vi "Build Actual View.vi"(5 "Encoder Counts Out":dbl[](array[numeric]), 7 "Speeds":dbl[](array[numeric]), 10 "Previous Actual":T5 {"Back Right"."Direction" scale format="%.3f"; "Back Right"."Velocity" format="%.2f"; "Back Left"."Direction" scale format="%.3f"; "Back Left"."Velocity" format="%.2f"; "Front Left"."Direction" scale format="%.3f"; "Front Left"."Velocity" format="%.2f"; "Front Right"."Direction" scale format="%.3f"; "Front Right"."Velocity" format="%.2f"}, 11 "Swerve Set":T1 {"Back Right"."Angle" scale format="%.3f"; "Back Right"."Velocity" scale=-1.0..1.0 scale format="%.1f"; "Back Left"."Angle" scale format="%.3f"; "Back Left"."Velocity" scale=-1.0..1.0 scale format="%.1f"; "Front Left"."Angle" scale format="%.3f"; "Front Left"."Velocity" scale=-1.0..1.0 scale format="%.1f"; "Front Right"."Angle" scale format="%.3f"; "Front Right"."Velocity" scale=-1.0..1.0 scale format="%.1f"}) -> (3 "Swerve Data out":T5 {"Back Right"."Direction" scale format="%.3f"; "Back Right"."Velocity" format="%.2f"; "Back Left"."Direction" scale format="%.3f"; "Back Left"."Velocity" format="%.2f"; "Front Left"."Direction" scale format="%.3f"; "Front Left"."Velocity" format="%.2f"; "Front Right"."Direction" scale format="%.3f"; "Front Right"."Velocity" format="%.2f"})   [LabVIEW 2020, in "SwerveDrive_ACT.lvlib"]
uses:
  SwerveDrive_ACT.lvlib
  Shared Code/TypeDefs/Cluster_Swerve Actual Settings.ctl
  Shared Code/TypeDefs/Cluster_Module Actual Settings.ctl
  Shared Code/TypeDefs/Dial_Actual Direction.ctl
  Shared Code/TypeDefs/Cluster_Swerve 4 Steer and Velocity.ctl
  Shared Code/TypeDefs/Cluster_Module Velocity-Direction-Rotations.ctl
  Shared Code/TypeDefs/Level_Velocity plus-minus 1.ctl
  Shared Code/TypeDefs/Dial_Compase heading unit circle CCW positive.ctl
panel:
  # "\"Front\" of Robot"
  # "Right Hand Rule"
  # "X"
  # "+CCW"
  # "Y"
  # "(0,0)"
  # "\"Front\" of Robot"
  # "X"
  # "+CCW"
  # "Y"
  # "(0,0)"
  # "\"Front\" of Robot"
  # "X"
  # "+CCW"
  # "Y"
  # "(0,0)"
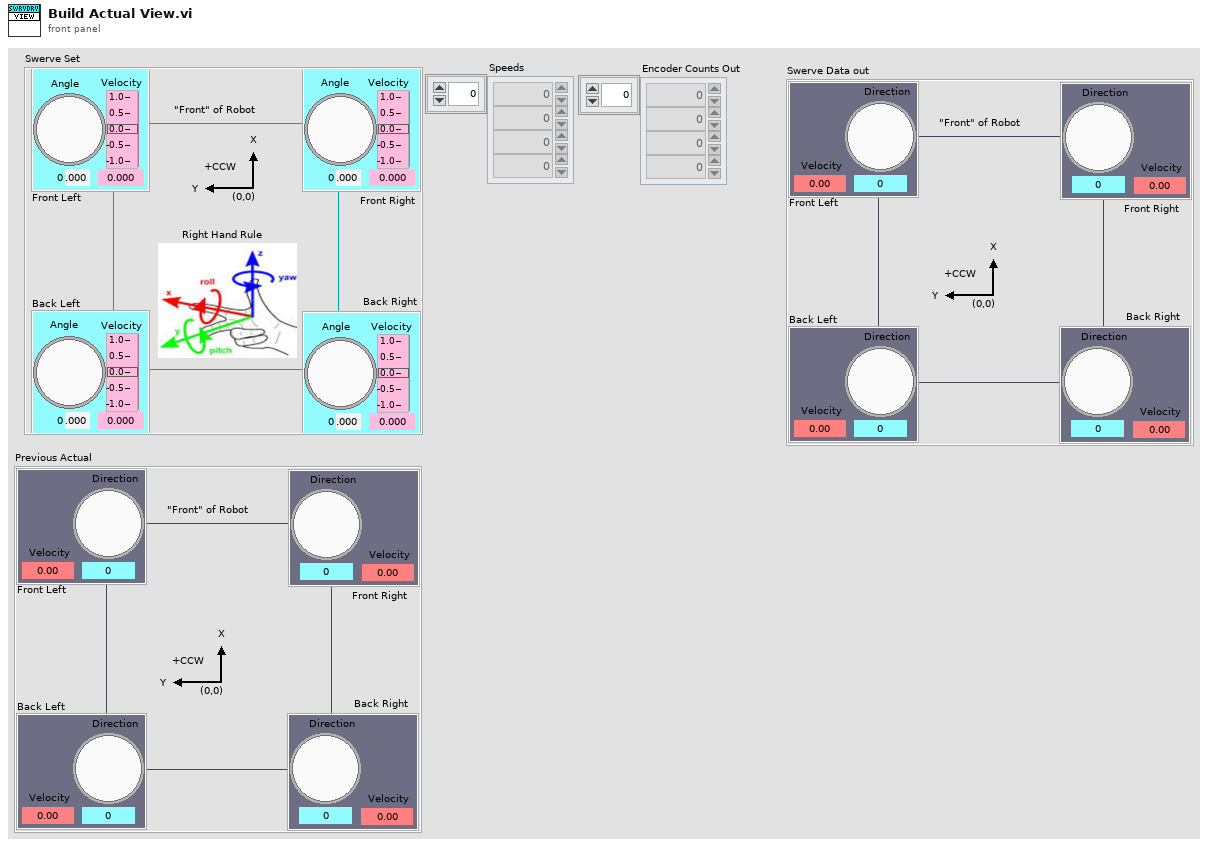
[diagram p1: front panel]
types:
  T1 = typedef "Cluster_Swerve 4 Steer and Velocity.ctl" = cluster{"Front Right":T2, "Front Left":T2, "Back Left":T2, "Back Right":T2}
  T2 = typedef "Cluster_Module Velocity-Direction-Rotations.ctl" = cluster{"Velocity":T3, "Angle":T4, "Rotations Count":dbl}
  T3 = typedef "Level_Velocity plus-minus 1.ctl" = dbl
  T4 = typedef "Dial_Compase heading unit circle CCW positive.ctl" = dbl
  T5 = typedef "Cluster_Swerve Actual Settings.ctl" = cluster{"Front Right":T6, "Front Left":T6, "Back Left":T6, "Back Right":T6}
  T6 = typedef "Cluster_Module Actual Settings.ctl" = cluster{"Velocity":dbl, "Direction":T7, "Encoder":dbl}
  T7 = typedef "Dial_Actual Direction.ctl" = dbl
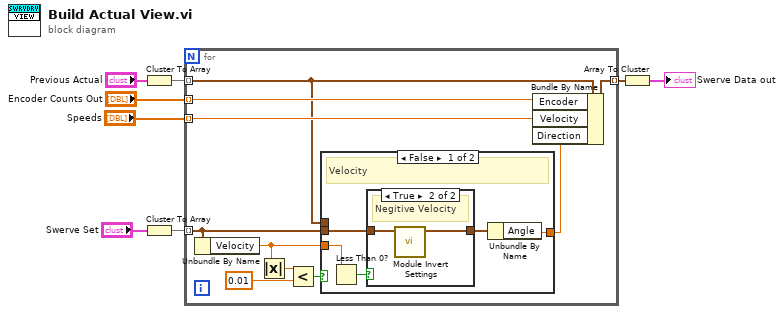
[diagram p0: block diagram]
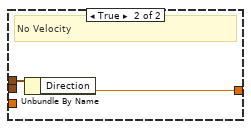
[diagram p3: hidden frame]
diagram:
  n1 = Cluster To Array(cluster="Previous Actual") -> (array=w6:T6[])
  n2 = Cluster To Array(cluster="Swerve Set") -> (array=w5:T2[])
  n3 = for {
    tunnel: w6 -> [w12] mode=indexing
    tunnel: w5 -> [w10] mode=indexing
    tunnel: "Encoder Counts Out" -> [w18] mode=indexing
    tunnel: "Speeds" -> [w16] mode=indexing
    tunnel: [w17] -> w2 mode=indexing
    n4 = Unbundle By Name(w10) -> ("Velocity"=w9:T3)
    n5 = Absolute Value(x=w9) -> (abs(x)=w15:T3)
    n6 = Less?(x=w15, y=T3 0.01) -> (x < y?=w13:bool)
    n7 = case shown="False" w13 {
      tunnel: w12 -> [_ w28]
      tunnel: [w19 w27] -> w11
      tunnel: w10 -> [w21 _]
      tunnel: w9 -> [w23 _]
      frame False {
        # "Velocity"
        n8 = Less Than 0?(x=w23) -> (x < 0?=w22:bool)
        n9 = case shown="True" w22 {
          tunnel: w21 -> [w24 w26]
          tunnel: [w24 w25] -> w20
          frame False {
            # "Positive Veloctiy"
          }
          frame True {
            # "Negitive Velocity"
            n10 = call "Module Invert Settings.vi"("Setting"=w26) -> ("Inverted Setting Out"=w25:T2)  [unwired: 10 in]
          }
        }
        n11 = Unbundle By Name(w20) -> ("Angle"=w19:T4)
      }
      frame True {
        # "No Velocity"
        n12 = Unbundle By Name(w28) -> ("Direction"=w27:T7)
      }
    }
    n13 = Bundle By Name(cluster=w12, "Encoder"=w18, "Velocity"=w16, "Direction"=w11) -> (w17:T6)
  }
  n14 = Array To Cluster(array=w2) -> (cluster=→"Swerve Data out":cluster{"[0]":T6, "[1]":T6, "[2]":T6, "[3]":T6})
